vi "nettest-snd.vi"() -> ()   [LabVIEW 2024]
uses:
  <vilib>/Utility/tcp.llb/UDP Multicast Read-Write Open.vi
panel:
  out "unsigned 32bit integer":u32
  out "length":i32
  in  "Array":T1(array[cluster])
  out "current time":timestamp
  out "Numeric":i32
  out "可能的網卡IP位置":string
  out "error out":errorcluster
  in  "stop":bool
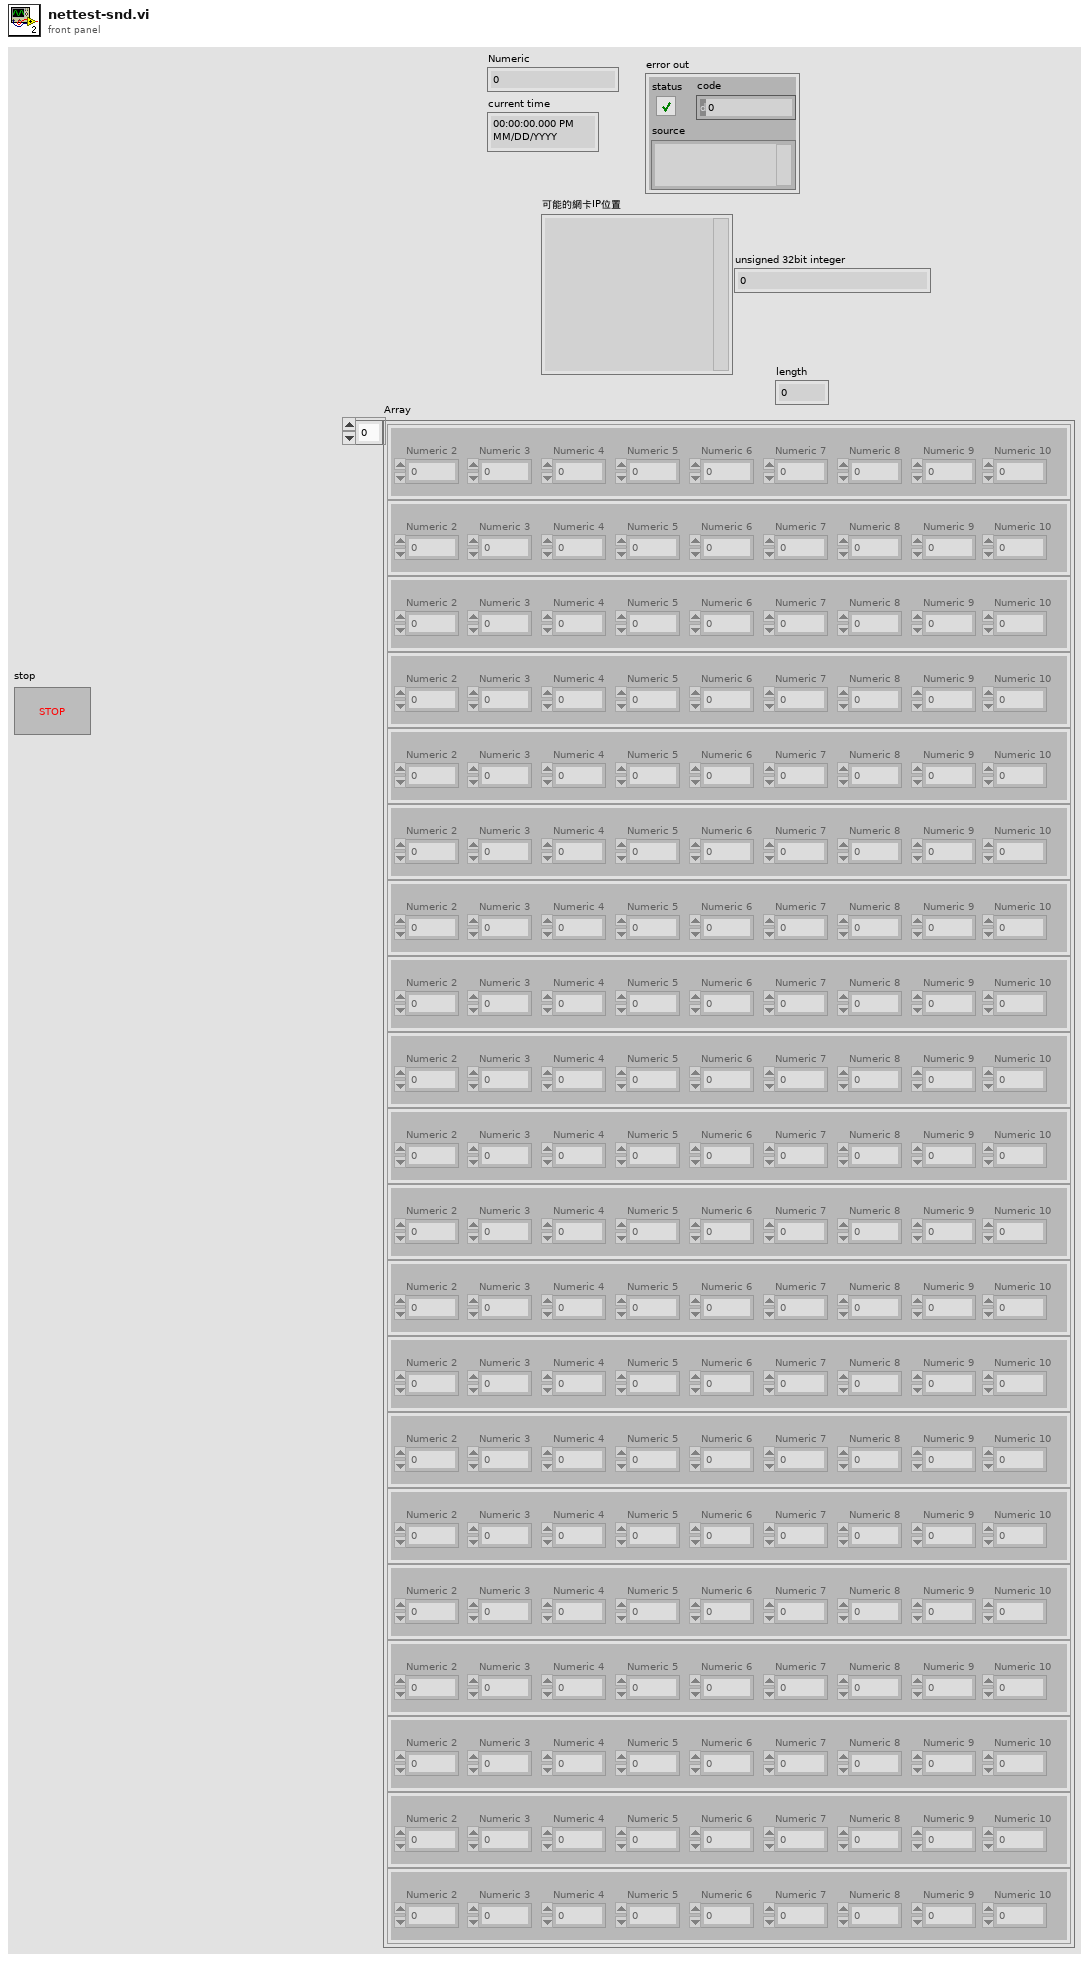
[diagram p1: front panel]
types:
  T1 = cluster{"Numeric 2":dbl, "Numeric 3":dbl, "Numeric 4":dbl, "Numeric 5":dbl, "Numeric 6":dbl, "Numeric 7":dbl, "Numeric 8":dbl, "Numeric 9":dbl, "Numeric 10":dbl}[]
  T2 = cluster{"Numeric 2":i16, "Numeric 3":i16, "Numeric 4":i16, "Numeric 5":i16, "Numeric 6":i16, "Numeric 7":i16, "Numeric 8":i16, "Numeric 9":i16, "Numeric 10":i16}[]
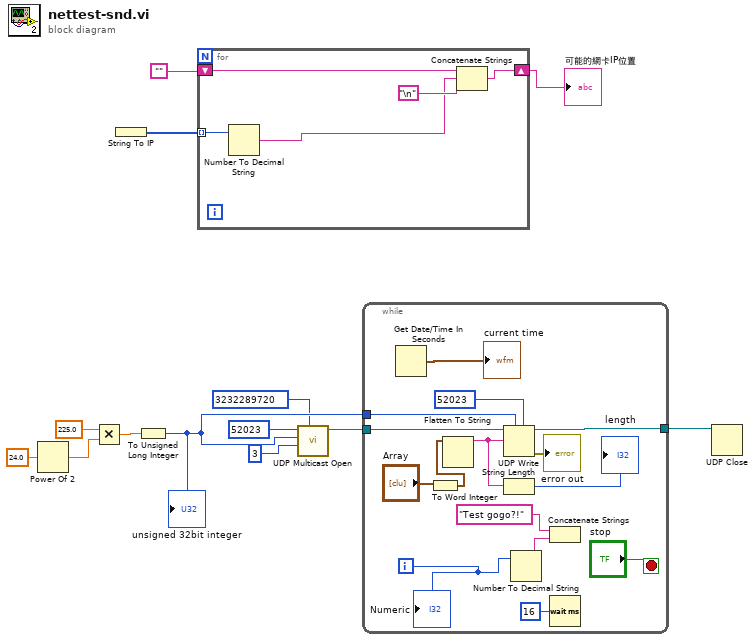
[diagram p0: block diagram]
diagram:
  n1 = Power Of 2(x=24.0) -> (2^x=w8:dbl)
  n2 = Multiply(x=225.0, y=w8) -> (x*y=w10:dbl)
  n3 = String To IP() -> (0:w2:u32[])  [unwired: 1 in]
  n4 = To Unsigned Long Integer(number=w10) -> (unsigned 32bit integer=w5:u32)
  "unsigned 32bit integer" <- w5
  n5 = for {
    shift-right: [w17] -> w3
    shift-left: "" -> [w18]
    tunnel: w2 -> [w15] mode=indexing
    n6 = Number To Decimal String(number=w15) -> (decimal integer string=w14:string)  [unwired: 1 in]
    n7 = Concatenate Strings(w18, w14, "\n") -> (w17:string)
  }
  "可能的網卡IP位置" <- w3
  n8 = call-poly <vilib>:"UDP Multicast Open.vi"("net address"=u32 3232289720, "time-to-live (1)"=u16 3, "multicast addr"=w5, "port"=u16 52023) -> ("connection ID"=w13:refnum<k16>)  [unwired: 5 in, 2 out]
  n9 = while {
    tunnel: w13 -> [w32]
    tunnel: [w31] -> w12
    tunnel: w5 -> [w30]
    i -> [w29]
    stop <- "stop" stop-if-true
    n10 = Get Date/Time In Seconds() -> (seconds since 1Jan1904=→"current time":timestamp)
    n11 = To Word Integer(number="Array") -> (16bit integer=w19:T2)
    n12 = Flatten To String(anything=w19) -> (data string=w22:string)  [unwired: 3 in, 2 out]
    n13 = UDP Write(address=w30, port or service name=u16 52023, connection ID=w32, data in=w22) -> (error out=→"error out":errorcluster, 3:w31:refnum<k16>)  [unwired: 2 in]
    n14 = String Length(string=w22) -> (length=→"length":i32)
    n15 = Number To Decimal String(number=w29) -> (decimal integer string=w28:string)  [unwired: 1 in]
    n16 = Concatenate Strings("Test gogo?!" ("data in"), w28) -> ()  [unwired: 1 out]
    n17 = Wait (ms)(milliseconds to wait=u32 16) -> ()  [unwired: 1 out]
    "Numeric" <- w29
  }
  n18 = UDP Close(connection ID=w12) -> ()  [unwired: 1 in, 2 out]
